vi "Process.vi"(8 "error in (no error)":errorcluster, 10 "Initialize CWC in":refnum<class "Initialize CWC.lvclass">, 11 "Architecture.lvlib:Thread.lvclass":refnum<class "Thread.lvclass">) -> (0 "error out":errorcluster, 1 "Stop?":bool, 3 "Architecture.lvlib:Thread.lvclass 2":refnum<class "Thread.lvclass">)   [LabVIEW 2012, in "Car Wash Controller.lvlib" / "Initialize CWC.lvclass"]
uses:
  Initialize CWC.lvclass
  Car Wash Controller/Car Wash Controller.lvclass
  Queue/Queue.lvclass
  Initialize VPS Msg/Initialize VPS.lvclass
  Initialize WDC Msg/Initialize WDC.lvclass
  Initialize Entry Console Msg/Initialize Entry Console.lvclass
  Thread/Thread.lvclass
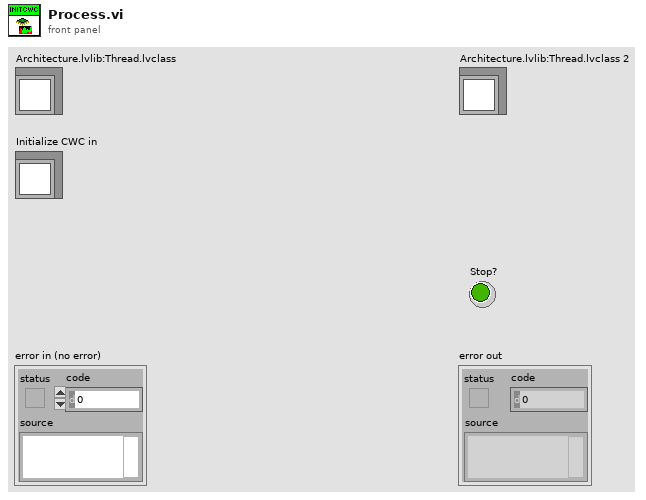
[diagram p1: front panel]
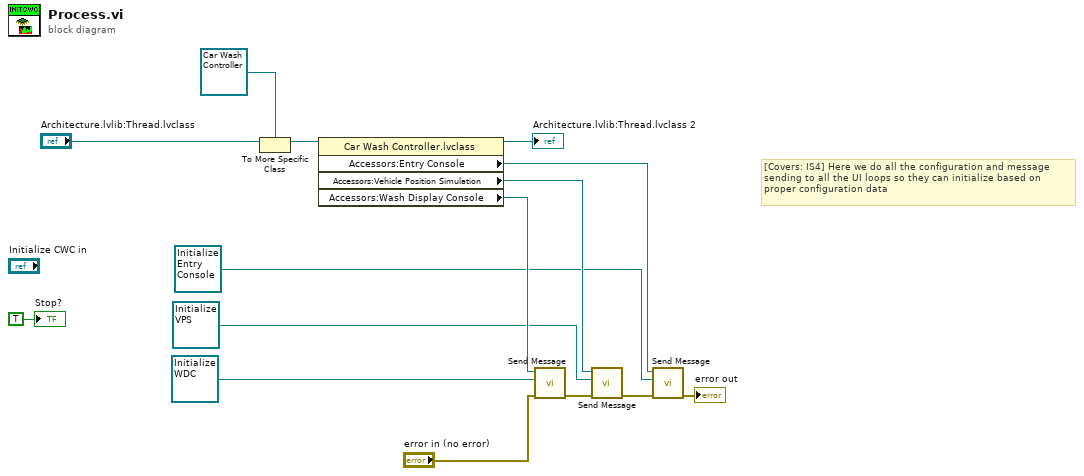
[diagram p0: block diagram]
diagram:
  # "[Covers: IS4] Here we do all the configuration and message\nsending to all the UI loops so they can initialize based on \nproper configuration data"
  n1 = To More Specific Class(target class=refnum<class "Car Wash Controller.lvclass"> refnum ("Car Wash Controller.lvlib:Car Wash Controller.lvclass"), reference="Architecture.lvlib:Thread.lvclass") -> (specific class reference=w13:refnum<class "Car Wash Controller.lvclass">)  [unwired: 1 in, 1 out]
  n2 = property class="Car Wash Controller.lvclass"(reference=w13) -> (reference out=→"Architecture.lvlib:Thread.lvclass 2":refnum<class "Car Wash Controller.lvclass">, "Accessors:Entry Console"=w10:refnum<class "Queue.lvclass">, "Accessors:Vehicle Position Simulation"=w11:refnum<class "Queue.lvclass">, "Accessors:Wash Display Console"=w12:refnum<class "Queue.lvclass">)  [unwired: 1 in, 1 out]
  n3 = call "Send Message.vi"("error in (no error)"="error in (no error)", "Architecture.lvlib:Message.lvclass"=refnum<class "Initialize WDC.lvclass"> refnum ("Wash Display Console.lvlib:Initialize WDC.lvclass"), "Queue in"=w12) -> ("error out"=w5:errorcluster)  [unwired: 7 in, 1 out]
  n4 = call "Send Message.vi"("error in (no error)"=w5, "Architecture.lvlib:Message.lvclass"=refnum<class "Initialize VPS.lvclass"> refnum ("Vehicle Position Simulation.lvlib:Initialize VPS.lvclass"), "Queue in"=w11) -> ("error out"=w6:errorcluster)  [unwired: 7 in, 1 out]
  n5 = call "Send Message.vi"("error in (no error)"=w6, "Architecture.lvlib:Message.lvclass"=refnum<class "Initialize Entry Console.lvclass"> refnum ("Entry Console.lvlib:Initialize Entry Console.lvclass"), "Queue in"=w10) -> ("error out"=→"error out":errorcluster)  [unwired: 7 in, 1 out]
  "Stop?" <- TRUE ("Stop?")
